vi "BRig_dataBlock_TPB_target.vi"() -> (2 "output_TPB_target":i32)   [LabVIEW 2014]
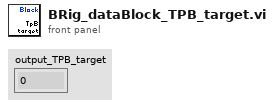
[diagram p1: front panel]
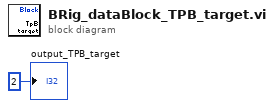
[diagram p0: block diagram]
diagram:
  "output_TPB_target" <- 2 ("output_iBlock")
